vi "J1939 Address Listen for Claim.vi"(0 "session in":refnum<k21>, 5 "ref in":T1, 7 "Requested Address":u8, 9 "timeout (0)":dbl, 11 "error in":errorcluster) -> (4 "session out":refnum<k21>, 6 "Conflict?":bool, 15 "error out":errorcluster)   [LabVIEW 2013, in "J1939.lvlib"]
uses:
  J1939.lvlib
  LUTs/J1939 Address Table Reference.ctl
  LUTs/J1939 Address Lookup Table Action.ctl
  LUTs/J1939 Address Lookup Table Data.ctl
  Frame Conversion/Convert CAN Arb ID to J1939 ID.vi
  <vilib>/xnet/xnet.llb/XNET Read (Frame CAN).vi
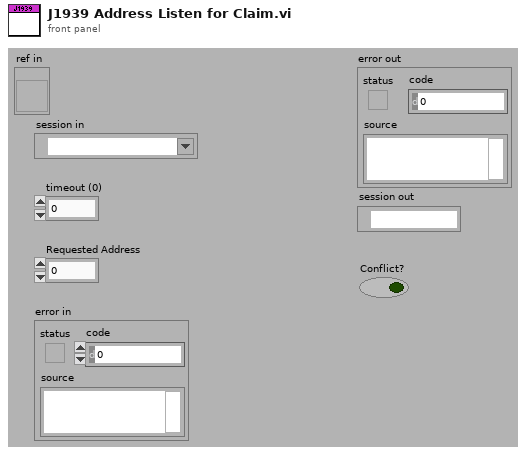
[diagram p1: front panel]
types:
  T1 = typedef "J1939.lvlib/J1939 Address Table Reference.ctl" = refnum<vi>
  T2 = typedef "J1939.lvlib/J1939 Address Lookup Table Data.ctl" = cluster{"Name":u8[], "Address":u8}
  T3 = typedef "J1939.lvlib/J1939 Address Lookup Table Action.ctl" = enum16{"Initialize", "Add", "Get", "Remove", "Get All"}
  T4 = typedef "XNET Frame CAN.ctl" = cluster{"timestamp":timestamp, "payload":u8[], "identifier":u32, "type":T5, "extended?":bool, "echo?":bool}
  T5 = typedef "XNET Frame Type CAN.ctl" = u8
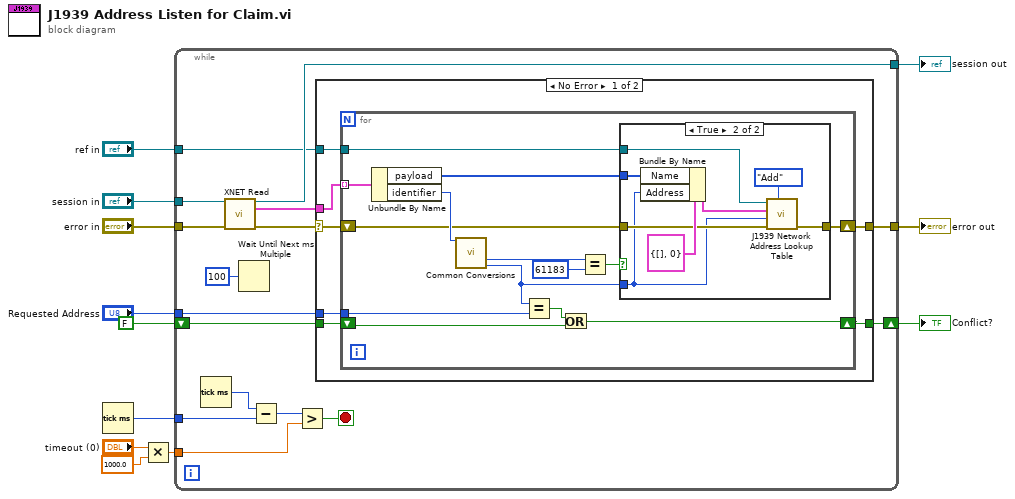
[diagram p0: block diagram]
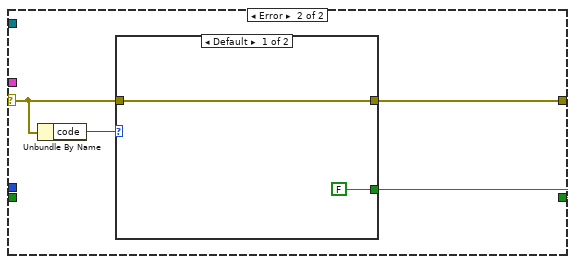
[diagram p3: hidden frame]
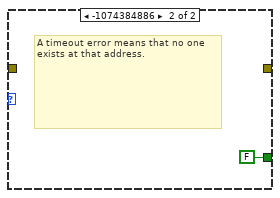
[diagram p4: hidden frame]
diagram:
  n1 = Tick Count (ms)() -> (millisecond timer value=w4:u32)
  n2 = Multiply(x="timeout (0)", y=1000.0) -> (x*y=w1:dbl)
  n3 = while {
    tunnel: "session in" -> [w28]
    tunnel: "Requested Address" -> [w27]
    tunnel: w1 -> [w14]
    tunnel: "error in" -> [w23]
    tunnel: [w22] -> w8
    tunnel: [w21] -> w7
    shift-right: [w25] -> w10
    shift-left: FALSE -> [w20]
    tunnel: "ref in" -> [w19]
    tunnel: w4 -> [w16]
    stop <- w13 stop-if-true
    n4 = Tick Count (ms)() -> (millisecond timer value=w17:u32)
    n5 = call-poly <vilib>:"XNET Read.vi"("session in"=w28, "error in (no error)"=w23) -> ("session out"=w21:refnum<k21>, "data"=w24:T4[], "error out"=w26:errorcluster)  [unwired: 11 out]
    n6 = Wait Until Next ms Multiple(millisecond multiple=u32 100) -> ()  [unwired: 1 out]
    n7 = Subtract(x=w17, y=w16) -> (x-y=w15:u32)
    n8 = Greater?(x=w15, y=w14) -> (0:w13:bool)
    n9 = case shown="No Error" w26 {
      selector: w26 -> [w31 w59]
      tunnel: w27 -> [w35 _]
      tunnel: w24 -> [w34 _]
      tunnel: [w33 w61] -> w25
      tunnel: [w30 w60] -> w22
      tunnel: w20 -> [w32 _]
      tunnel: w19 -> [w29 _]
      frame No Error {
        n10 = for {
          tunnel: w34 -> [w49] mode=indexing
          tunnel: w35 -> [w45]
          shift-right: [w39] -> w33
          shift-left: w32 -> [w40]
          shift-right: [w37] -> w30
          shift-left: w31 -> [w38]
          tunnel: w29 -> [w36]
          n11 = Unbundle By Name(w49) -> ("payload"=w42:u8[], "identifier"=w48:u32)
          n12 = call-poly "Common Conversions.vi"("Arb ID"=w48) -> ("PGN"=w47:u32, "Source Address"=w43:u8)  [unwired: 11 in, 2 out]
          n13 = Equal?(x=w43, y=w45) -> (x = y?=w41:bool)
          n14 = Or(x=w41, y=w40) -> (x .or. y?=w39:bool)
          n15 = Equal?(x=w47, y=u32 61183) -> (x = y?=w44:bool)
          n16 = case shown="True" w44 {
            tunnel: w43 -> [_ w51]
            tunnel: w42 -> [_ w57]
            tunnel: w38 -> [w50 w54]
            tunnel: [w50 w53] -> w37
            tunnel: w36 -> [_ w52]
            frame False {
            }
            frame True {
              n17 = Bundle By Name(cluster=T2 {"Name"=[], "Address"=0} ("Data"), "Name"=w57, "Address"=w51) -> (w55:T2)
              n18 = call "J1939 Network Address Lookup Table.vi"("Action"=J1939_Address_Lookup_Table_Action."Add", "error in (no error)"=w54, "Address"=w51, "Data"=w55, "ref in"=w52) -> ("error out"=w53:errorcluster)  [unwired: 3 in, 3 out]
            }
          }
        }
      }
      frame Error {
        n19 = Unbundle By Name(w59) -> ("code"=w62:i32)
        n20 = case shown="Default" w62 {
          tunnel: [FALSE FALSE] -> w61
          tunnel: [w63 _] -> w60
          tunnel: w59 -> [w63 _]
          frame Default {
          }
          frame -1074384886 {
            # "A timeout error means that no one exists at that address."
          }
        }
      }
    }
  }
  "Conflict?" <- w10
  "error out" <- w8
  "session out" <- w7
